vi "Read Arduino Temperature Controller.vi"(8 "Error In":errorcluster, 11 "VISA resource name":refnum<visa-resource-name>) -> (0 "Error Out":errorcluster, 1 "Control temperature":dbl, 2 "Sample temperature":dbl, 3 "VISA resource name out":refnum<visa-resource-name>, 4 "Power":dbl, 5 "Set point":dbl)   [LabVIEW 2019]
panel:
  out "IDN":string
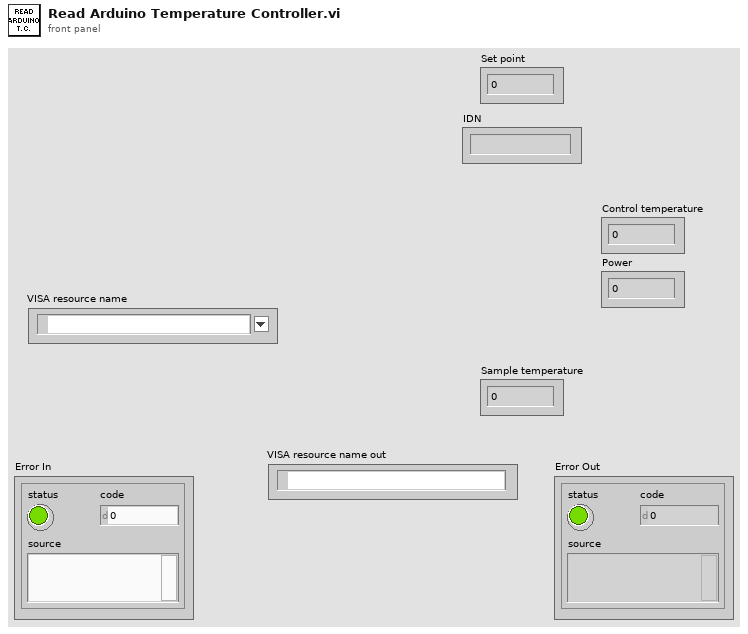
[diagram p1: front panel]
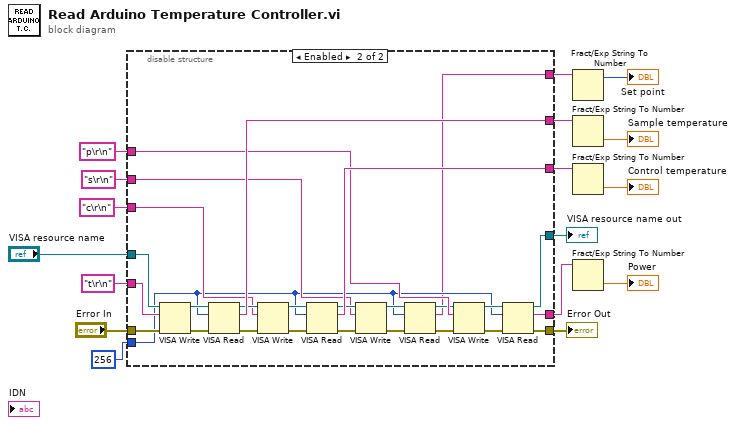
[diagram p0: block diagram]
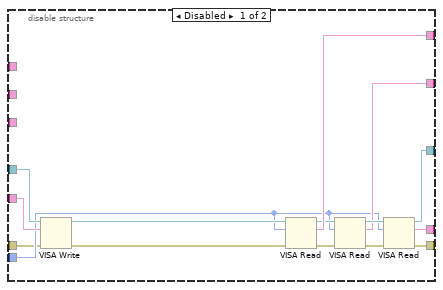
[diagram p2: hidden frame]
diagram:
  n1 = disable-structure shown="Enabled" {
    disable-tunnel: "VISA resource name" -> [w32 w59]
    disable-tunnel: "t\r\n" ("write buffer") -> [w31 w58]
    disable-tunnel: [w28 w55] -> w15
    disable-tunnel: [w23 w54] -> w14
    disable-tunnel: [w22 w53] -> w5
    disable-tunnel: u32 256 ("byte count") -> [w21 w34]
    disable-tunnel: "Error In" -> [w20 w52]
    disable-tunnel: [w19 w51] -> w11
    disable-tunnel: [w18 w50] -> w10
    disable-tunnel: "c\r\n" ("write buffer") -> [_ w43]
    disable-tunnel: "p\r\n" ("write buffer") -> [_ w42]
    disable-tunnel: "s\r\n" ("write buffer") -> [_ w35]
    disable-tunnel: [_ w33] -> w6
    frame Disabled {
      n2 = VISA Write(VISA resource name=w32, write buffer=w31, error in (no error)=w20) -> (VISA resource name out=w30:refnum<visa-resource-name>, error out=w29:errorcluster)  [unwired: 1 out]
      n3 = VISA Read(VISA resource name=w30, byte count=w21, error in (no error)=w29) -> (VISA resource name out=w27:refnum<visa-resource-name>, read buffer=w28:string, error out=w25:errorcluster)  [unwired: 1 out]
      n4 = VISA Read(VISA resource name=w27, byte count=w21, error in (no error)=w25) -> (VISA resource name out=w26:refnum<visa-resource-name>, read buffer=w23:string, error out=w24:errorcluster)  [unwired: 1 out]
      n5 = VISA Read(VISA resource name=w26, byte count=w21, error in (no error)=w24) -> (VISA resource name out=w18:refnum<visa-resource-name>, read buffer=w22:string, error out=w19:errorcluster)  [unwired: 1 out]
    }
    frame Enabled {
      n6 = VISA Write(VISA resource name=w59, write buffer=w58, error in (no error)=w52) -> (VISA resource name out=w57:refnum<visa-resource-name>, error out=w56:errorcluster)  [unwired: 1 out]
      n7 = VISA Read(VISA resource name=w57, byte count=w34, error in (no error)=w56) -> (VISA resource name out=w47:refnum<visa-resource-name>, read buffer=w55:string, error out=w49:errorcluster)  [unwired: 1 out]
      n8 = VISA Write(VISA resource name=w47, write buffer=w43, error in (no error)=w49) -> (VISA resource name out=w46:refnum<visa-resource-name>, error out=w48:errorcluster)  [unwired: 1 out]
      n9 = VISA Read(VISA resource name=w46, byte count=w34, error in (no error)=w48) -> (VISA resource name out=w39:refnum<visa-resource-name>, read buffer=w54:string, error out=w37:errorcluster)  [unwired: 1 out]
      n10 = VISA Write(VISA resource name=w39, write buffer=w35, error in (no error)=w37) -> (VISA resource name out=w40:refnum<visa-resource-name>, error out=w41:errorcluster)  [unwired: 1 out]
      n11 = VISA Read(VISA resource name=w40, byte count=w34, error in (no error)=w41) -> (VISA resource name out=w38:refnum<visa-resource-name>, read buffer=w33:string, error out=w36:errorcluster)  [unwired: 1 out]
      n12 = VISA Write(VISA resource name=w38, write buffer=w42, error in (no error)=w36) -> (VISA resource name out=w45:refnum<visa-resource-name>, error out=w44:errorcluster)  [unwired: 1 out]
      n13 = VISA Read(VISA resource name=w45, byte count=w34, error in (no error)=w44) -> (VISA resource name out=w50:refnum<visa-resource-name>, read buffer=w53:string, error out=w51:errorcluster)  [unwired: 1 out]
    }
  }
  "VISA resource name out" <- w10
  "Error Out" <- w11
  n14 = Fract/Exp String To Number(string=w6) -> (offset past number=→"Set point":i32)  [unwired: 3 in, 1 out]
  n15 = Fract/Exp String To Number(string=w15) -> (number=→"Sample temperature":dbl)  [unwired: 3 in, 1 out]
  n16 = Fract/Exp String To Number(string=w14) -> (number=→"Control temperature":dbl)  [unwired: 3 in, 1 out]
  n17 = Fract/Exp String To Number(string=w5) -> (number=→"Power":dbl)  [unwired: 3 in, 1 out]
